vi "Get Event Handlers Dict.vi"(8 "error in (no error)":errorcluster, 10 "Event In":refnum<class "Event.lvclass">, 11 "Controller in":refnum<class "Controller.lvclass">) -> (0 "error out":errorcluster, 1 "Event Handlers Dict":variant, 2 "Event out":refnum<class "Event.lvclass">, 3 "Event Found":bool, 5 "Event ID":string)   [LabVIEW 2023, in "MVC Actors.lvlib" / "Controller.lvclass"]
uses:
  Controller.lvclass
  Event/Event.lvclass
  Controller.lvclass/Controller.ctl
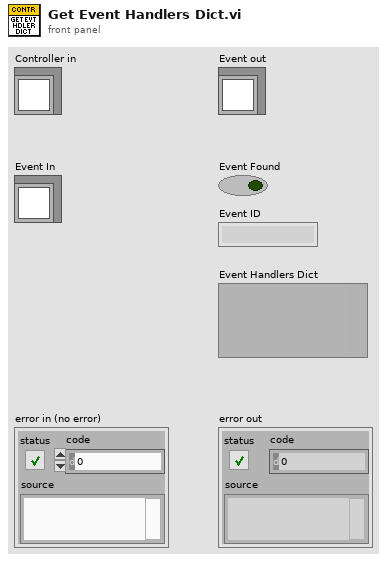
[diagram p1: front panel]
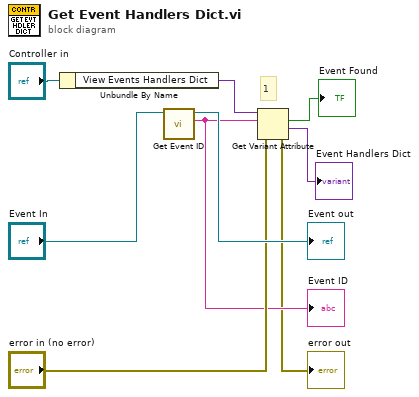
[diagram p0: block diagram]
diagram:
  # "1"
  n1 = Unbundle By Name("Controller in") -> ("View Events Handlers Dict"=w2:variant)
  n2 = call-dynamic "Get Event ID.vi"("Event in"="Event In") -> ("Event ID"=w7:string, "Event out"=→"Event out":refnum<class "Event.lvclass">)  [unwired: 8 in, 1 out]
  "Event ID" <- w7
  n3 = Get Variant Attribute(Variant=w2, name=w7, error in="error in (no error)") -> (found=→"Event Found":bool, value=→"Event Handlers Dict":variant, error out=→"error out":errorcluster)  [unwired: 1 in, 1 out]
